vi "Add.vi"(8 "error in (no error)":errorcluster, 9 "parent tag":string, 10 "Destinations in":refnum<class "IB_Destination.lvclass">[](array[class]), 11 "IB_Destination in":refnum<class "IB_Destination.lvclass">) -> (0 "error out":errorcluster, 1 "duplicate?":bool, 2 "Destinations out":refnum<class "IB_Destination.lvclass">[](array[class]), 3 "IB_Destination out":refnum<class "IB_Destination.lvclass">)   [LabVIEW 2020, in "IB_Destination.lvclass"]
uses:
  <vilib>/AppBuilder/IB_Classes/Destination/IB_Destination.lvclass
  <vilib>/AppBuilder/IB_Classes/Destination/IB_Destination.lvclass/IB_Destination.ctl
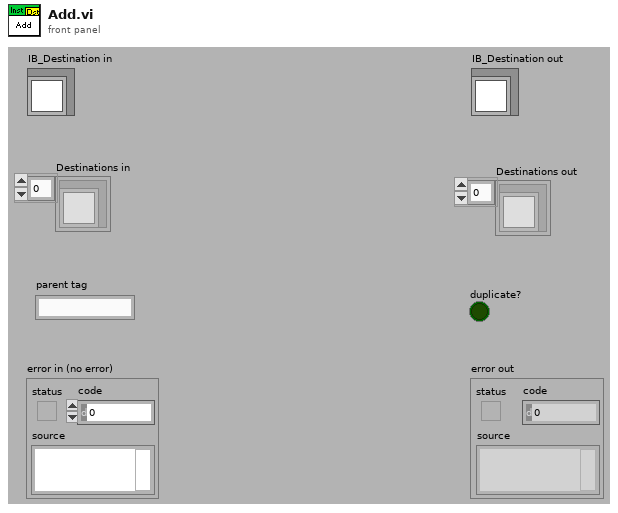
[diagram p1: front panel]
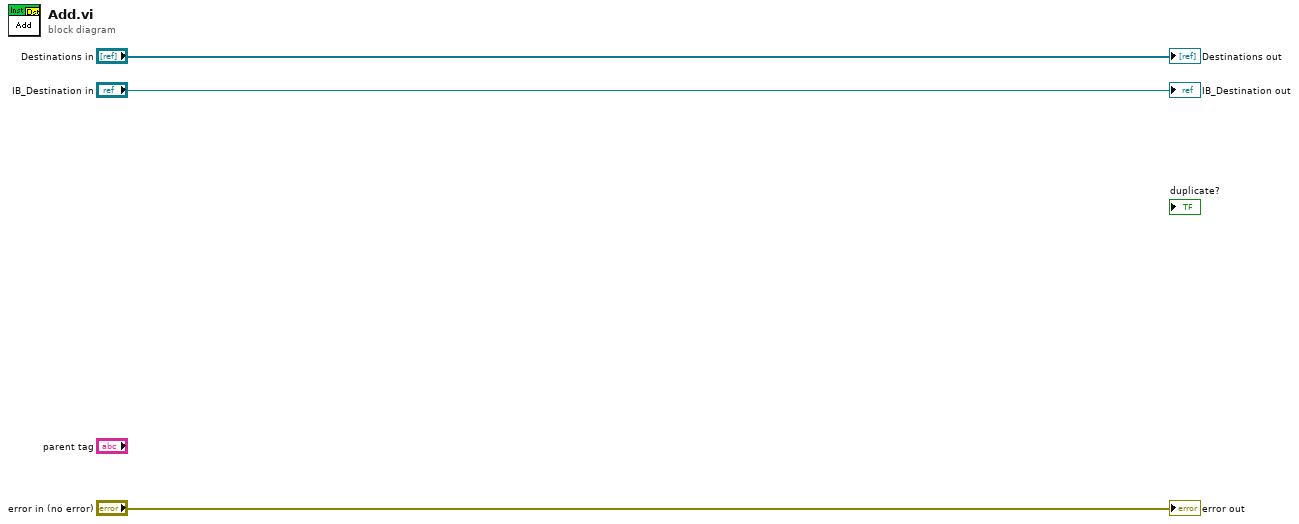
[diagram p0: block diagram]
diagram:
  "error out" <- "error in (no error)"
  "IB_Destination out" <- "IB_Destination in"
  "Destinations out" <- "Destinations in"
